vi "Rinocloud_HTTP_delete_metadata_field.vi"(5 "error in (no error)":errorcluster, 7 "field":string, 8 "ID":string) -> (0 "error out":errorcluster, 3 "Status":T1={"headers"="", "body"="", "ID"="", "Saved"=TRUE})   [LabVIEW 2011, in "Rinocloud Library.lvlib"]
uses:
  Rinocloud Library.lvlib
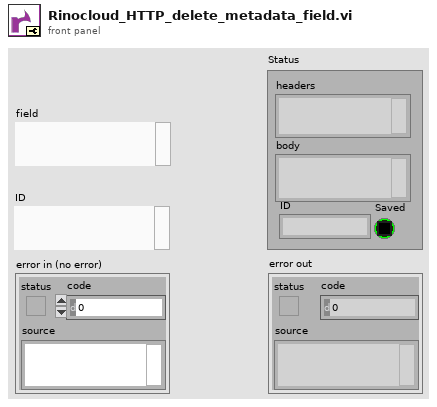
[diagram p1: front panel]
types:
  T1 = cluster{"headers":string, "body":string, "ID":string, "Saved":bool}
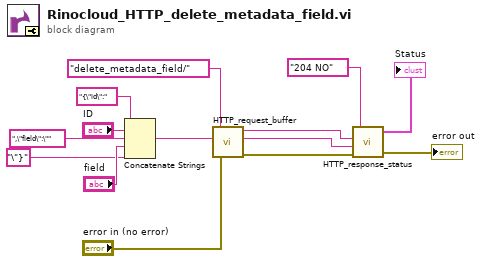
[diagram p0: block diagram]
diagram:
  n1 = Concatenate Strings("{\"id\":" ("string"), "ID", ",\"field\":\"" ("string"), "field", "\"}" ("string")) -> (w9:string)
  n2 = call "HTTP_request_buffer.vi"("error in (no error)"="error in (no error)", "JSON payload"=w9, "Endpoint"="delete_metadata_field/") -> ("error out"=w12:errorcluster, "body"=w5:string, "headers"=w6:string)  [unwired: 2 in]
  n3 = call "HTTP_response_status.vi"("error in (no error)"=w12, "body"=w5, "headers"=w6, "HTTP status"="204 NO") -> ("error out"=→"error out":errorcluster, "Status"=→"Status":T1)  [unwired: 1 in]
